vi "Writer Page.vi"(8 "error in (no error)":errorcluster, 11 "Node Ptr":T3 format="%.0x") -> (0 "error out":errorcluster)   [LabVIEW 2015, in "DDS Custom Device System Explorer.lvlib"]
uses:
  DDS Custom Device System Explorer.lvlib
  <vilib>/NI Veristand/Custom Device API/Custom Device Item Ref.ctl
  Shared/MyTopic ComplexType.ctl
  Shared/key Enum.ctl
  Shared/Constants.vi
  <vilib>/NI Veristand/Custom Device API/Set Item Property (String).vi
  <vilib>/NI VeriStand/Custom Device API/Custom Device API.lvlib
  Shared/DDS Custom Device Shared.lvlib
panel:
  in  "Default Key":T1
  in  "Topic Default Values":T2={"I32_Num"=0, "I64_Num"=0, "U16_Num"=0, "Sgl_Array"=[0.0, 0.0, 0.0, 0.0], "innercluster"={"Sgl_Num"=0.0, "Boolean"=FALSE}}
  in  "Force Unbounded String?":bool
  in  "Force Array Mapping?":bool
  in  "Data Writer QoS Profile":string
  in  "Domain Participant QoS Profile":string
  in  "Type Name":string
  in  "Domain id":u32
  in  "Topic Name":string
  in  "SHDocVw.IWebBrowser":refnum<k7>(container)
  in  "General Header":cluster{"Section Name":string}={"Section Name"="General Custom Device Settings"}
  in  "Description":string
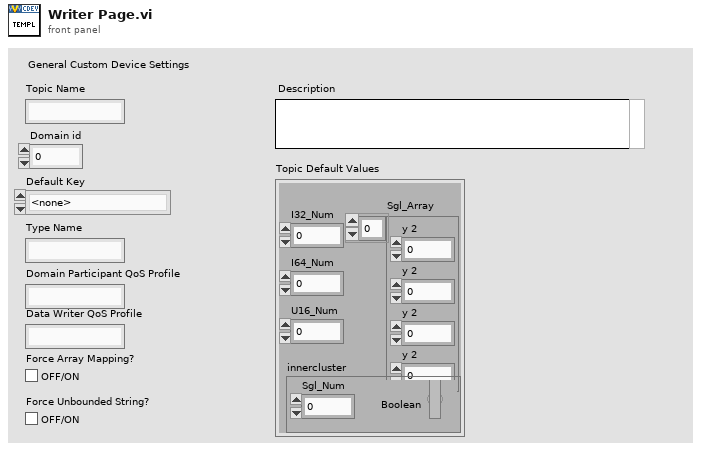
[diagram p1: front panel]
types:
  T1 = typedef "DDS Custom Device Shared.lvlib/key Enum.ctl" = enum16{"<none>", "I32_Num", "I64_Num", "U16_Num", "innercluster.Sgl_Num", "innercluster.Boolean"}
  T2 = typedef "DDS Custom Device Shared.lvlib/MyTopic ComplexType.ctl" = cluster{"I32_Num":i32, "I64_Num":i64, "U16_Num":u16, "Sgl_Array":sgl[], "innercluster":cluster{"Sgl_Num":sgl, "Boolean":bool}}
  T3 = typedef "Custom Device API.lvlib/Custom Device Item Ref.ctl" = u64
  T4 = typedef "Custom Device API.lvlib/Custom Device Item Info.ctl" = cluster{"Name":string, "Is Channel":bool, "GUID":string, "Is Waveform":bool}
  T5 = typedef "DDS Custom Device Shared.lvlib/WriterReaderConfiguration.ctl" = cluster{"Topic Name":string, "Domain Id":u32, "Advanced Configuration":T6}
  T6 = typedef "DDS Custom Device Shared.lvlib/Advanced DDS Configuration.ctl" = cluster{"typeName":string, "key Name":T1, "domainParticipantQoSProfile":string, "dataWriterQoSProfile":string, "forceArrayMapping?":bool, "forceUnboundedString?":bool, "forceExclusiveReader?":bool, "forceRead? (only ExclusiveReader)":bool, "ContentFilteredTopic Info":T7}
  T7 = typedef "LVDDS_library.lvlib/RTI DDS ContentFilteredTopic Info.ctl" = cluster{"Filter Type":string, "ContentFilteredTopic Name":string, "Filter Expression":string}
  T8 = typedef "Custom Device API.lvlib/Custom Device Commands.ctl" = enum16{"Default", "Item renamed", "Shutdown", "Dynamic button pressed"}
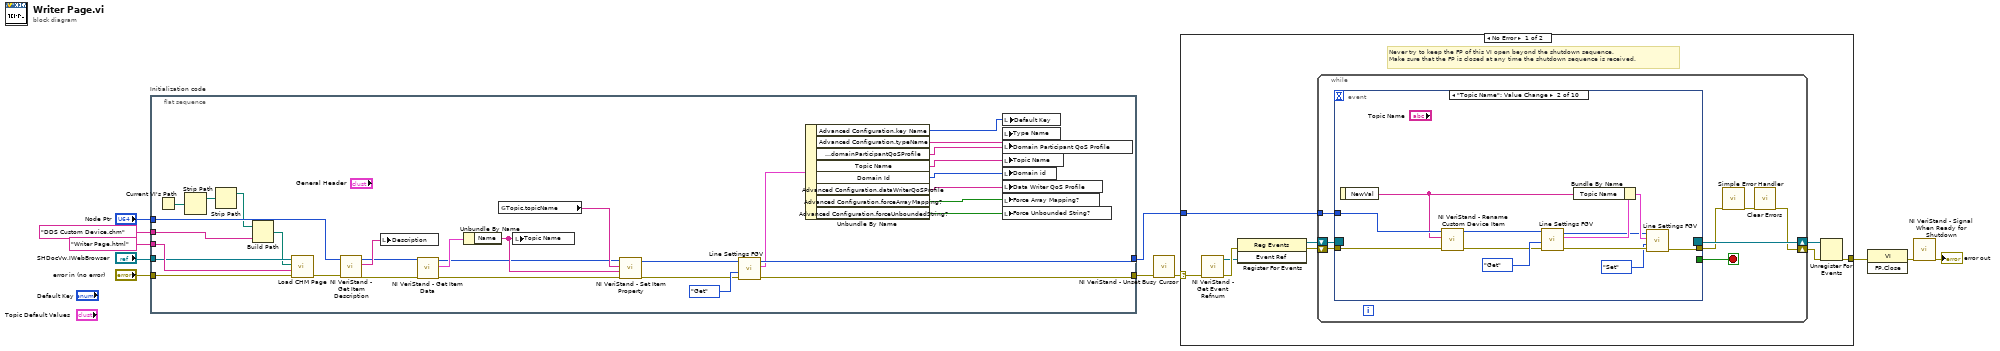
[diagram p0: block diagram]
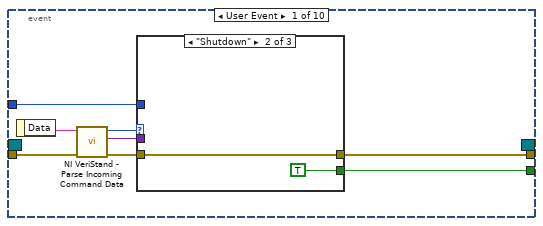
[diagram p2: hidden frame]
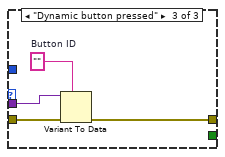
[diagram p4: hidden frame]
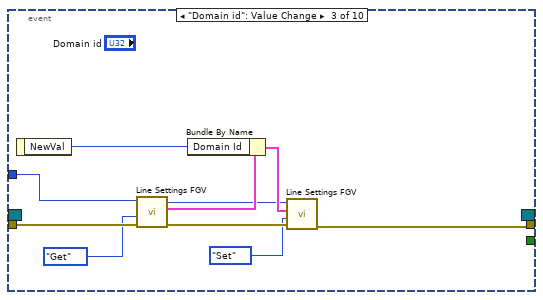
[diagram p5: hidden frame]
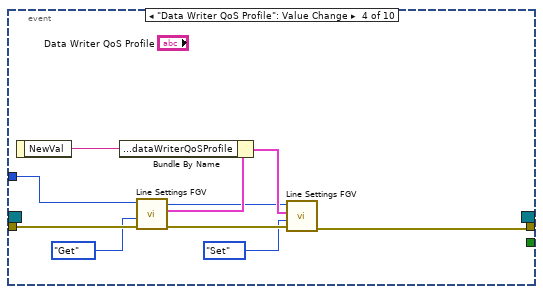
[diagram p6: hidden frame]
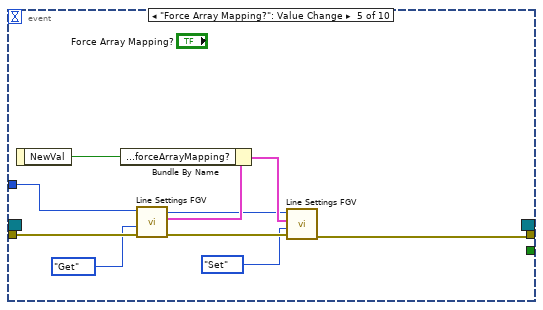
[diagram p7: hidden frame]
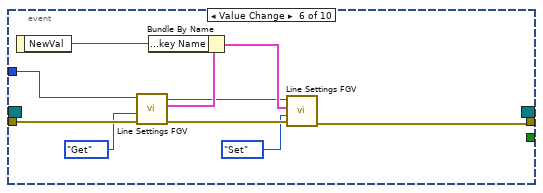
[diagram p8: hidden frame]
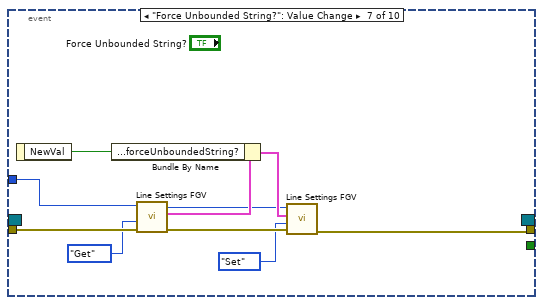
[diagram p9: hidden frame]
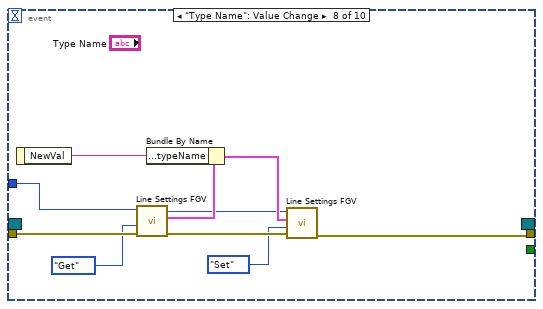
[diagram p10: hidden frame]
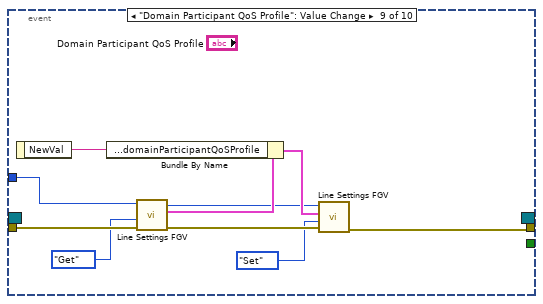
[diagram p11: hidden frame]
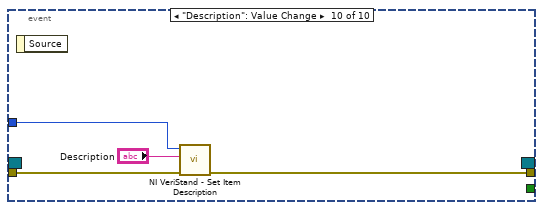
[diagram p12: hidden frame]
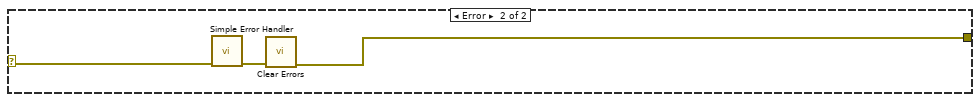
[diagram p13: hidden frame]
diagram:
  n1 = flat-sequence "Initialization code" {
    tunnel: "error in (no error)" -> [w41]
    tunnel: "Node Ptr" -> [w43]
    tunnel: [w36] -> w7
    tunnel: [w35] -> w4
    tunnel: "SHDocVw.IWebBrowser" -> [w39]
    tunnel: "Writer Page.html" ("HTML File") -> [w40]
    tunnel: "DDS Custom Device.chm" ("CD_CHM_FileName") -> [w20]
    frame #0 {
      n2 = Current VI's Path() -> (path=w23:path)
      n3 = Strip Path(path=w23) -> (stripped path=w22:path)  [unwired: 1 out]
      n4 = Strip Path(path=w22) -> (stripped path=w21:path)  [unwired: 1 out]
      n5 = Build Path(base path=w21, name or relative path=w20) -> (appended path=w19:path)
      n6 = call <vilib>:"Load CHM Page.vi"("error in (no error)"=w41, "HTML File"=w40, "Main CHM File Path"=w19, "Web Browser Reference"=w39) -> ("error out"=w42:errorcluster)  [unwired: 7 in]
      n7 = call <vilib>:"NI VeriStand - Get Item Description.vi"("error in (no error)"=w42, "Item Ref in"=w43) -> ("error out"=w25:errorcluster, "Description"=w38:string, "Item Ref out"=w26:T3)  [unwired: 7 out]
      n8 = local write "Description"(w38) -> ()
      n9 = call <vilib>:"NI VeriStand - Get Item Data.vi"("error in (no error)"=w25, "Item Ref in"=w26) -> ("error out"=w15:errorcluster, "Item Info"=w24:T4, "Item Ref out"=w14:T3)  [unwired: 6 in, 1 out]
      n10 = Unbundle By Name(w24) -> ("Name"=w16:string)
      n11 = global read "Constants.vi" "Topic.topicName"() -> (w17:string)
      n12 = local write "Topic Name"(w16) -> ()
      n13 = call-poly <vilib>:"NI VeriStand - Set Item Property.vi"("error in (no error)"=w15, "Value"=w16, "Property Name"=w17, "Item Ref in"=w14) -> ("error out"=w13:errorcluster, "Item Ref out"=w12:T3)  [unwired: 5 in, 1 out]
      n14 = call "Line Settings FGV.vi"("error in (no error)"=w13, "Get/Set"=enum16{"Set", "Get"}."Get", "Item Ref in"=w12) -> ("error out"=w36:errorcluster, "Line"=w34:T5, "Item Ref out"=w35:T3)  [unwired: 6 in]
      n15 = Unbundle By Name(w34) -> ("Advanced Configuration.key Name"=w18:T1, "Advanced Configuration.typeName"=w33:string, "Advanced Configuration.domainParticipantQoSProfile"=w32:string, "Topic Name"=w31:string, "Domain Id"=w30:u32, "Advanced Configuration.dataWriterQoSProfile"=w29:string, "Advanced Configuration.forceArrayMapping?"=w28:bool, "Advanced Configuration.forceUnboundedString?"=w27:bool)
      n16 = local write "Type Name"(w33) -> ()
      n17 = local write "Domain Participant QoS Profile"(w32) -> ()
      n18 = local write "Topic Name"(w31) -> ()
      n19 = local write "Domain id"(w30) -> ()
      n20 = local write "Data Writer QoS Profile"(w29) -> ()
      n21 = local write "Force Array Mapping?"(w28) -> ()
      n22 = local write "Force Unbounded String?"(w27) -> ()
      n23 = local write "Default Key"(w18) -> ()
    }
  }
  n24 = call <vilib>:"NI VeriStand - Unset Busy Cursor.vi"("error in (no error)"=w7) -> ("error out"=w6:errorcluster)  [unwired: 10 out]
  n25 = case shown="No Error" w6 {
    selector: w6 -> [w44 w164]
    tunnel: [w49 w162] -> w11
    tunnel: w4 -> [w45 _]
    frame No Error {
      # "Never try to keep the FP of this VI open beyond the shutdown sequence.\nMake sure that the FP is closed at any time the shutdown sequence is received."
      n26 = call <vilib>:"NI VeriStand - Get Event Refnum.vi"("error in (no error)"=w44) -> ("error out"=w52:errorcluster, "Event Ref"=w48:refnum<user-event>)  [unwired: 9 out]
      n27 = register-events(error in=w52, w48) -> (reference out=w46:refnum<event-registration>, error out=w47:errorcluster)  [unwired: 1 in]
      n28 = while {
        tunnel: w45 -> [w56]
        shift-right: [w53] -> w50
        shift-left: w47 -> [w59]
        shift-right: [w60] -> w51
        shift-left: w46 -> [w58]
        stop <- w57 stop-if-true
        n29 = event shown="[1] \"Topic Name\": Value Change" {
          selector: w58 -> [_ _ _ _ _ _ _ _ _ _]
          dyn-events: [_ _ _ _ _ _ _ _ _ _] -> w60
          timeout: _ -> [_ _ _ _ _ _ _ _ _ _]
          tunnel: w59 -> [w68 w79 w97 w107 w117 w127 w137 w147 w157 w160]
          tunnel: [w64 _ _ _ _ _ _ _ _ _] -> w57
          tunnel: [w63 w82 w89 w99 w109 w119 w129 w139 w149 w159] -> w55
          tunnel: w56 -> [w62 w80 w96 w106 w116 w126 w136 w146 w156 w161]
          event User Event {
            n30 = event-data() -> ("Data"=w67:string)  [unwired: 1 out]
            n31 = call <vilib>:"NI VeriStand - Parse Incoming Command Data.vi"("error in (no error)"=w68, "Incoming data"=w67) -> ("error out"=w66:errorcluster, "Outgoing data"=w61:variant, "Action"=w65:T8)  [unwired: 7 out]
            n32 = case shown="\"Shutdown\"" w65 {
              tunnel: w66 -> [w69 w70 w75]
              tunnel: [_ TRUE _] -> w64
              tunnel: [w69 w70 w72] -> w63
              tunnel: w62 -> [_ _ _]
              tunnel: w61 -> [_ _ w74]
              frame "Default", Default {
              }
              frame "Shutdown" {
              }
              frame "Dynamic button pressed" {
                w73 = ""  # Button ID
                n33 = Variant To Data(error in=w75, type=w73, Variant=w74) -> (error out=w72:errorcluster)  [unwired: 1 out]
              }
            }
          }
          event "Topic Name": Value Change {
            n34 = event-data() -> ("NewVal"=w76:string)  [unwired: 1 out]
            n35 = call <vilib>:"NI VeriStand - Rename Custom Device Item.vi"("error in (no error)"=w79, "New Name"=w76, "Item Ref in"=w80) -> ("error out"=w78:errorcluster, "Item Ref out"=w77:T3)  [unwired: 6 in, 1 out]
            n36 = call "Line Settings FGV.vi"("error in (no error)"=w78, "Get/Set"=enum16{"Set", "Get"}."Get", "Item Ref in"=w77) -> ("error out"=w86:errorcluster, "Line"=w85:T5, "Item Ref out"=w83:T3)  [unwired: 6 in]
            n37 = Bundle By Name(cluster=w85, "Topic Name"=w76) -> (w84:T5)
            n38 = call "Line Settings FGV.vi"("error in (no error)"=w86, "Get/Set"=enum16{"Set", "Get"}."Set", "Line"=w84, "Item Ref in"=w83) -> ("error out"=w82:errorcluster)  [unwired: 5 in, 2 out]
          }
          event "Domain id": Value Change {
            n39 = event-data() -> ("NewVal"=w92:u32)  [unwired: 1 out]
            n40 = call "Line Settings FGV.vi"("error in (no error)"=w97, "Get/Set"=enum16{"Set", "Get"}."Get", "Item Ref in"=w96) -> ("error out"=w94:errorcluster, "Line"=w93:T5, "Item Ref out"=w90:T3)  [unwired: 6 in]
            n41 = Bundle By Name(cluster=w93, "Domain Id"=w92) -> (w91:T5)
            n42 = call "Line Settings FGV.vi"("error in (no error)"=w94, "Get/Set"=enum16{"Set", "Get"}."Set", "Line"=w91, "Item Ref in"=w90) -> ("error out"=w89:errorcluster)  [unwired: 5 in, 2 out]
          }
          event "Data Writer QoS Profile": Value Change {
            n43 = event-data() -> ("NewVal"=w102:string)  [unwired: 1 out]
            n44 = call "Line Settings FGV.vi"("error in (no error)"=w107, "Get/Set"=enum16{"Set", "Get"}."Get", "Item Ref in"=w106) -> ("error out"=w104:errorcluster, "Line"=w103:T5, "Item Ref out"=w100:T3)  [unwired: 6 in]
            n45 = Bundle By Name(cluster=w103, "Advanced Configuration.dataWriterQoSProfile"=w102) -> (w101:T5)
            n46 = call "Line Settings FGV.vi"("error in (no error)"=w104, "Get/Set"=enum16{"Set", "Get"}."Set", "Line"=w101, "Item Ref in"=w100) -> ("error out"=w99:errorcluster)  [unwired: 5 in, 2 out]
          }
          event "Force Array Mapping?": Value Change {
            n47 = event-data() -> ("NewVal"=w112:bool)  [unwired: 1 out]
            n48 = call "Line Settings FGV.vi"("error in (no error)"=w117, "Get/Set"=enum16{"Set", "Get"}."Get", "Item Ref in"=w116) -> ("error out"=w114:errorcluster, "Line"=w113:T5, "Item Ref out"=w110:T3)  [unwired: 6 in]
            n49 = Bundle By Name(cluster=w113, "Advanced Configuration.forceArrayMapping?"=w112) -> (w111:T5)
            n50 = call "Line Settings FGV.vi"("error in (no error)"=w114, "Get/Set"=enum16{"Set", "Get"}."Set", "Line"=w111, "Item Ref in"=w110) -> ("error out"=w109:errorcluster)  [unwired: 5 in, 2 out]
          }
          event Value Change {
            n51 = event-data() -> ("NewVal"=w122:T1)  [unwired: 1 out]
            n52 = call "Line Settings FGV.vi"("error in (no error)"=w127, "Get/Set"=enum16{"Set", "Get"}."Get", "Item Ref in"=w126) -> ("error out"=w124:errorcluster, "Line"=w123:T5, "Item Ref out"=w120:T3)  [unwired: 6 in]
            n53 = Bundle By Name(cluster=w123, "Advanced Configuration.key Name"=w122) -> (w121:T5)
            n54 = call "Line Settings FGV.vi"("error in (no error)"=w124, "Get/Set"=enum16{"Set", "Get"}."Set", "Line"=w121, "Item Ref in"=w120) -> ("error out"=w119:errorcluster)  [unwired: 5 in, 2 out]
          }
          event "Force Unbounded String?": Value Change {
            n55 = event-data() -> ("NewVal"=w132:bool)  [unwired: 1 out]
            n56 = call "Line Settings FGV.vi"("error in (no error)"=w137, "Get/Set"=enum16{"Set", "Get"}."Get", "Item Ref in"=w136) -> ("error out"=w134:errorcluster, "Line"=w133:T5, "Item Ref out"=w130:T3)  [unwired: 6 in]
            n57 = Bundle By Name(cluster=w133, "Advanced Configuration.forceUnboundedString?"=w132) -> (w131:T5)
            n58 = call "Line Settings FGV.vi"("error in (no error)"=w134, "Get/Set"=enum16{"Set", "Get"}."Set", "Line"=w131, "Item Ref in"=w130) -> ("error out"=w129:errorcluster)  [unwired: 5 in, 2 out]
          }
          event "Type Name": Value Change {
            n59 = event-data() -> ("NewVal"=w142:string)  [unwired: 1 out]
            n60 = call "Line Settings FGV.vi"("error in (no error)"=w147, "Get/Set"=enum16{"Set", "Get"}."Get", "Item Ref in"=w146) -> ("error out"=w144:errorcluster, "Line"=w143:T5, "Item Ref out"=w140:T3)  [unwired: 6 in]
            n61 = Bundle By Name(cluster=w143, "Advanced Configuration.typeName"=w142) -> (w141:T5)
            n62 = call "Line Settings FGV.vi"("error in (no error)"=w144, "Get/Set"=enum16{"Set", "Get"}."Set", "Line"=w141, "Item Ref in"=w140) -> ("error out"=w139:errorcluster)  [unwired: 5 in, 2 out]
          }
          event "Domain Participant QoS Profile": Value Change {
            n63 = event-data() -> ("NewVal"=w152:string)  [unwired: 1 out]
            n64 = call "Line Settings FGV.vi"("error in (no error)"=w157, "Get/Set"=enum16{"Set", "Get"}."Get", "Item Ref in"=w156) -> ("error out"=w154:errorcluster, "Line"=w153:T5, "Item Ref out"=w150:T3)  [unwired: 6 in]
            n65 = Bundle By Name(cluster=w153, "Advanced Configuration.domainParticipantQoSProfile"=w152) -> (w151:T5)
            n66 = call "Line Settings FGV.vi"("error in (no error)"=w154, "Get/Set"=enum16{"Set", "Get"}."Set", "Line"=w151, "Item Ref in"=w150) -> ("error out"=w149:errorcluster)  [unwired: 5 in, 2 out]
          }
          event "Description": Value Change {
            n67 = event-data() -> ()  [unwired: 2 out]
            n68 = call <vilib>:"NI VeriStand - Set Item Description.vi"("error in (no error)"=w160, "Description"="Description", "Item Ref in"=w161) -> ("error out"=w159:errorcluster)  [unwired: 8 out]
          }
        }
        n69 = call <vilib>:"Simple Error Handler.vi"("error in (no error)"=w55) -> ("error out"=w54:errorcluster)  [unwired: 1 in, 7 out]
        n70 = call <vilib>:"Clear Errors.vi"("error in (no error)"=w54) -> ("error out"=w53:errorcluster)  [unwired: 1 in, 5 out]
      }
      n71 = Unregister For Events(event registration refnum=w51, error in=w50) -> (error out=w49:errorcluster)
    }
    frame Error {
      n72 = call <vilib>:"Simple Error Handler.vi"("error in (no error)"=w164) -> ("error out"=w163:errorcluster)  [unwired: 1 in, 7 out]
      n73 = call <vilib>:"Clear Errors.vi"("error in (no error)"=w163) -> ("error out"=w162:errorcluster)  [unwired: 1 in, 5 out]
    }
  }
  n74 = invoke class="VI" method="FP.Close"(error in=w11) -> (error out=w10:errorcluster)  [unwired: 2 in, 2 out]
  n75 = call <vilib>:"NI VeriStand - Signal When Ready for Shutdown.vi"("error in (no error)"=w10) -> ("error out"=→"error out":errorcluster)  [unwired: 10 out]
